vi "DWF MSO Query Digital Edge Trigger.vi"(0 "Instrument Handle In":u32, 11 "Error In":errorcluster caption="Error In (no error)", 12 "Trigger Instance":i32(ring) caption="Trigger Instance (A)" items=["A", "B"]) -> (4 "Instrument Handle Out":u32, 6 "Trigger Source":string, 8 "Trigger Slope":i32(ring) items=["Rising", "Falling", "Either"], 15 "Error Out":errorcluster)   [LabVIEW 2015, in "DigilentWF.lvlib"]
doc: "Indicates the digital trigger configuration of the specified instance."
uses:
  <vilib>/DigilentWF/DigilentWF.lvlib
  dwf.dll
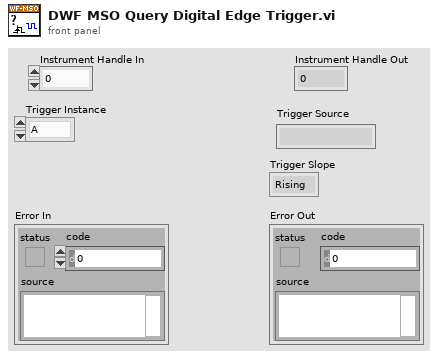
[diagram p1: front panel]
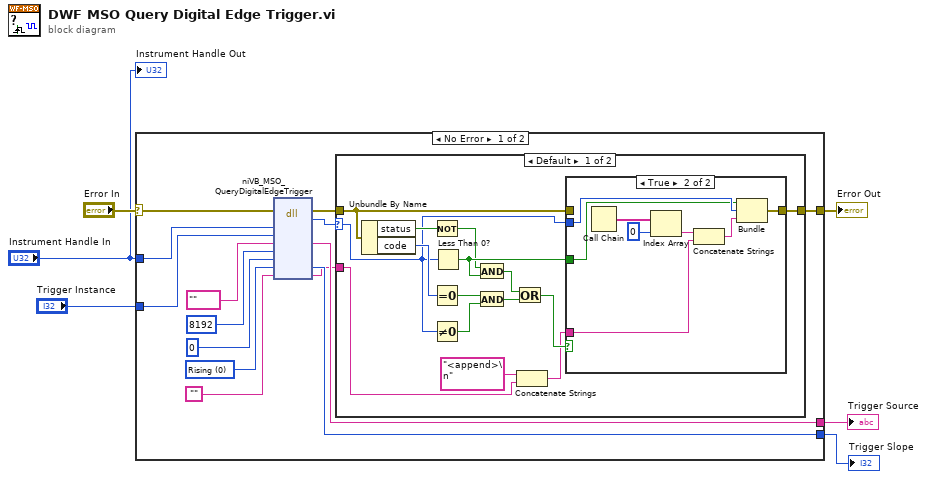
[diagram p0: block diagram]
diagram:
  n1 = case "outter_case" shown="No Error" "Error In" {
    selector: "Error In" -> [w20 w46]
    tunnel: [w17 w46] -> w5
    tunnel: "Instrument Handle In" -> [w16 _]
    tunnel: "Trigger Instance" -> [w15 _]
    tunnel: [w12 _] -> w1
    tunnel: [w11 _] -> w2
    frame No Error {
      w13 = 0 items=["Rising", "Falling", "Either"] ("Trigger Slope")
      n2 = dll-call lib="dwf.*" fn="niVB_MSO_QueryDigitalEdgeTrigger"(error in=w20, "InstrumentHandle"=w16, "TriggerInstance"=w15, "TriggerSource"=tag "" ("Trigger Source"), "cTriggerSource"=8192, "pTriggerSource"=0, "TriggerSlope"=w13, "szError"="") -> (error out=w19:errorcluster, "return type"=w18:i32, "TriggerSource"=w12:string, "TriggerSlope"=w11:i32, "szError"=w10:string)  [unwired: 6 in, 1 out]
      n3 = case "inner_case" shown="Default" w18 {
        selector: w18 -> [w25 _]
        tunnel: w19 -> [w26 w45]
        tunnel: [w22 w45] -> w17
        tunnel: w10 -> [w21 _]
        frame Default {
          n4 = Unbundle By Name(w26) -> ("status"=w30:bool, "code"=w34:i32)
          n5 = Not(x=w30) -> (.not. x?=w33:bool)
          n6 = Equal To 0?(x=w34) -> (x = 0?=w29:bool)
          n7 = Not Equal To 0?(x=w25) -> (x != 0?=w32:bool)
          n8 = Less Than 0?(x=w25) -> (x < 0?=w35:bool)
          n9 = And(x=w33, y=w35) -> (x .and. y?=w31:bool)
          n10 = And(x=w29, y=w32) -> (x .and. y?=w28:bool)
          n11 = Or(x=w31, y=w28) -> (x .or. y?=w27:bool)
          n12 = Concatenate Strings("<append>\n" ("string"), w21) -> (w24:string)
          n13 = case shown="True" w27 {
            tunnel: [w36 w43] -> w22
            tunnel: w25 -> [_ w42]
            tunnel: w35 -> [_ w41]
            tunnel: w26 -> [w36 _]
            tunnel: w24 -> [_ w37]
            frame False {
            }
            frame True {
              n14 = Call Chain() -> (call chain=w40:string[])
              n15 = Index Array(array=w40, index=0) -> (element=w39:string)
              n16 = Concatenate Strings(w39, w37) -> (w44:string)
              n17 = Bundle(w41, "return type"=w42, w44) -> (w43:cluster{bool, "return type":i32, string})  [unwired: 1 out]
            }
          }
        }
        frame 0 {
        }
      }
    }
    frame Error {
    }
  }
  "Error Out" <- w5
  "Trigger Slope" <- w2
  "Trigger Source" <- w1
  "Instrument Handle Out" <- "Instrument Handle In"
